vi "Find Best Solution In Best Solutions Array.vi"(11 "Best Solution Array":T1[](array[typedef])) -> (3 "Best Solution":T1)   [LabVIEW 2013]
uses:
  Classes/GA_Class/Controls/Solution_GA.ctl
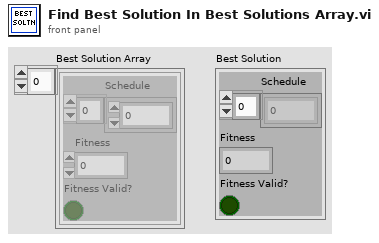
[diagram p1: front panel]
types:
  T1 = typedef "Solution_GA.ctl" = cluster{"Schedule":u16[], "Fitness":u16, "Fitness Valid?":bool}
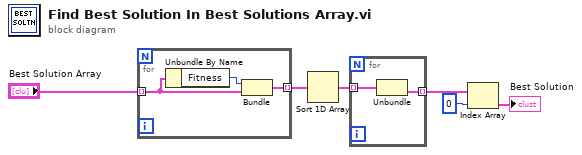
[diagram p0: block diagram]
diagram:
  n1 = for {
    tunnel: "Best Solution Array" -> [w8] mode=indexing
    tunnel: [w7] -> w5 mode=indexing
    n2 = Unbundle By Name(w8) -> ("Fitness"=w9:u16)
    n3 = Bundle("Fitness"=w9, "Solution"=w8) -> (w7:cluster{"Fitness":u16, "Solution":T1})  [unwired: 1 in]
  }
  n4 = Sort 1D Array(array=w5) -> (sorted array=w4:cluster{"Fitness":u16, "Solution":T1}[])
  n5 = for {
    tunnel: w4 -> [w11] mode=indexing
    tunnel: [w10] -> w3 mode=indexing
    n6 = Unbundle(w11) -> ("Solution"=w10:T1)  [unwired: 1 out]
  }
  n7 = Index Array(array=w3, index=0) -> (element=→"Best Solution":T1)
